vi "Is Set.vi"(8 "error in (no error)":errorcluster, 11 "Raw Message in":refnum<class "Raw Message.lvclass">) -> (0 "error out":errorcluster, 2 "Is Set":bool, 3 "Raw Message out":refnum<class "Raw Message.lvclass">)   [LabVIEW 2020, in "Protobuf RAW.lvlib" / "Raw Message.lvclass"]
uses:
  Raw Message.lvclass
  Raw Message.lvclass/Raw Message.ctl
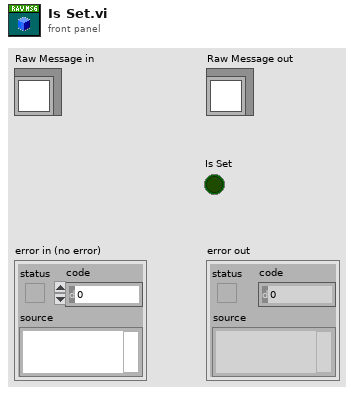
[diagram p1: front panel]
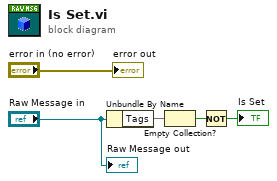
[diagram p0: block diagram]
diagram:
  n1 = Unbundle By Name("Raw Message in") -> ("Tags"=w4:map{u32, refnum<class "Basic Type.lvclass">[]})
  n2 = Empty Collection?(1:w4) -> (0:w3:bool)
  n3 = Not(x=w3) -> (.not. x?=→"Is Set":bool)
  "error out" <- "error in (no error)"
  "Raw Message out" <- "Raw Message in"
